vi "perform.vi"(8 "error in (no error)":errorcluster, 10 "Sensor Data":T2 {"Robot Heading" format="%05.1f"; "Wind Direction" format="%05.1f"}, 11 "MissionQueue in":refnum<class "MissionQueue.lvclass">) -> (0 "error out":errorcluster, 1 "Valid?":bool, 2 "Desired Location":T1, 3 "MissionQueue out":refnum<class "MissionQueue.lvclass">)   [LabVIEW 2011, in "MissionQueue.lvclass"]
uses:
  MissionQueue.lvclass
  2-RIO/2 Typedefs/sensorData.ctl
  2-RIO/2 Typedefs/UTM Location.ctl
  2-RIO/2 Typedefs/heading.ctl
  Mission/Mission.lvclass
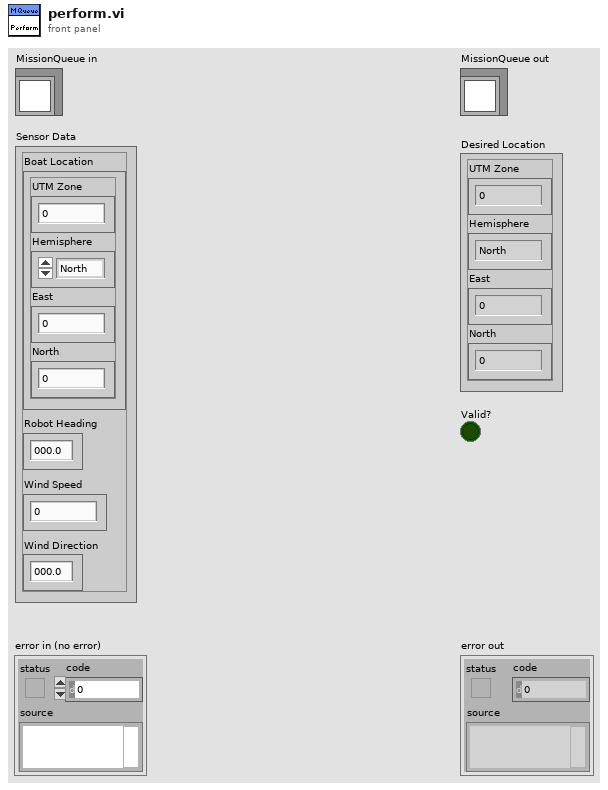
[diagram p1: front panel]
types:
  T1 = typedef "UTM Location.ctl" = cluster{"UTM Zone":dbl, "Hemisphere":enum16{"North", "South"}, "East":dbl, "North":dbl}
  T2 = typedef "sensorData.ctl" = cluster{"Boat Location":T1, "Robot Heading ":T3, "Wind Speed":dbl, "Wind Direction":T3}
  T3 = typedef "heading.ctl" = dbl
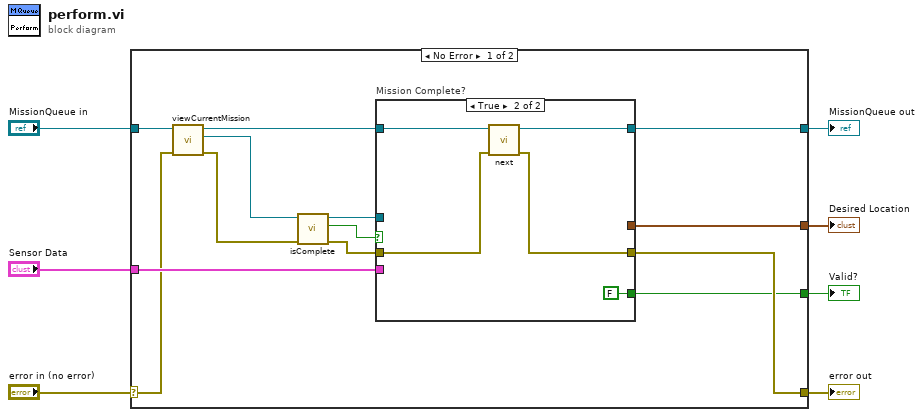
[diagram p0: block diagram]
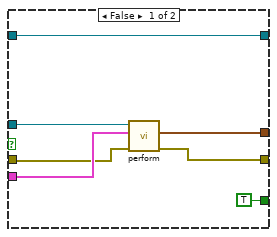
[diagram p2: hidden frame]
diagram:
  n1 = case shown="No Error" "error in (no error)" {
    selector: "error in (no error)" -> [w10 w34]
    tunnel: [w16 w34] -> w6
    tunnel: [w15 w33] -> w4
    tunnel: "MissionQueue in" -> [w12 w33]
    tunnel: "Sensor Data" -> [w18 _]
    tunnel: [w14 _] -> w2
    tunnel: [w13 _] -> w1
    frame No Error {
      n2 = call "viewCurrentMission.vi"("error in (no error)"=w10, "MissionQueue in"=w12) -> ("error out"=w9:errorcluster, "Mission.lvclass"=w8:refnum<class "Mission.lvclass">, "MissionQueue out"=w11:refnum<class "MissionQueue.lvclass">)  [unwired: 6 in, 1 out]
      n3 = call-dynamic "isComplete.vi"("error in (no error)"=w9, "Mission in"=w8) -> ("error out"=w17:errorcluster, "Mission Complete?"=w19:bool, "Mission out"=w20:refnum<class "Mission.lvclass">)  [unwired: 7 in]
      n4 = case "Mission Complete?" shown="True" w19 {
        tunnel: w20 -> [w25 _]
        tunnel: w18 -> [w27 _]
        tunnel: w17 -> [w26 w30]
        tunnel: [w24 w29] -> w16
        tunnel: w11 -> [w23 w32]
        tunnel: [w23 w31] -> w15
        tunnel: [w22 _] -> w14
        tunnel: [TRUE ("Valid?") FALSE ("Valid?")] -> w13
        frame False {
          n5 = call-dynamic "perform.vi"("error in (no error)"=w26, "Sensor Data"=w27, "Mission in"=w25) -> ("error out"=w24:errorcluster, "Desired Location"=w22:T1)  [unwired: 6 in, 1 out]
        }
        frame True {
          n6 = call "next.vi"("error in (no error)"=w30, "MissionQueue in"=w32) -> ("error out"=w29:errorcluster, "MissionQueue out"=w31:refnum<class "MissionQueue.lvclass">)  [unwired: 6 in, 2 out]
        }
      }
    }
    frame Error {
    }
  }
  "error out" <- w6
  "MissionQueue out" <- w4
  "Desired Location" <- w2
  "Valid?" <- w1
